vi "Set Logging Root.vi"(8 "error in (no error)":errorcluster, 10 "Logging Root":path, 11 "BasicEventLogger in":refnum<class "BasicEventLogger.lvclass">) -> (0 "error out":errorcluster, 3 "BasicEventLogger out":refnum<class "BasicEventLogger.lvclass">)   [LabVIEW 2020, in "Volatus.lvlib" / "BasicEventLogger.lvclass"]
uses:
  BasicEventLogger.lvclass
  BasicEventLogger.lvclass/BasicEventLogger.ctl
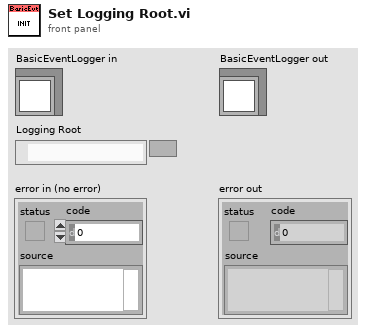
[diagram p1: front panel]
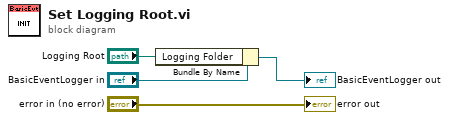
[diagram p0: block diagram]
diagram:
  n1 = Bundle By Name(cluster="BasicEventLogger in", "Logging Folder"="Logging Root") -> (→"BasicEventLogger out":refnum<class "BasicEventLogger.lvclass">)
  "error out" <- "error in (no error)"
